vi "GT Active Scheduler wSubset Standalone.vi"() -> ()   [LabVIEW 2013, in "Scheduler.lvclass"]
uses:
  Scheduler.lvclass
  OSSP_Problem.lvclass
  Operation Selection Rule from Subset to Schedule.ctl
  Prins FIFO Scheduler Methods and Controls/Controls/Prins FIFO Scheduler Result Cluster.ctl
  OSSP_Problem.lvclass/OSSP_Problem.ctl
  Operation to Machine Job Tuple.vi
  GT Find Subset of Operations.vi
  Select Operation to Schedule Based on Rule.vi
  OSSP_Problem_Class/Getters/Read Due Dates.vi
  <vilib>/dlg_ctls.llb/Space Constant.vi
  <vilib>/Heliosphere Research LLC/Advanced Plotting Toolkit/api_core/New.vi
  <vilib>/Heliosphere Research LLC/Advanced Plotting Toolkit/api_annotations/XLabel.vi
  <vilib>/Heliosphere Research LLC/Advanced Plotting Toolkit/api_figure/YTicks.vi
  <vilib>/Heliosphere Research LLC/Advanced Plotting Toolkit/api_figure/Grids.vi
  <vilib>/Heliosphere Research LLC/Advanced Plotting Toolkit/api_core/View.vi
  <vilib>/Heliosphere Research LLC/Advanced Plotting Toolkit/api_core/Close.vi
  <vilib>/Heliosphere Research LLC/Advanced Plotting Toolkit/api_figure/Limits.vi
  <vilib>/Heliosphere Research LLC/Advanced Plotting Toolkit/api_annotations/Rectangle.vi
  <vilib>/Heliosphere Research LLC/Advanced Plotting Toolkit/api_annotations/Text.vi
panel:
  out "Graph Out":picture
  out "Ordered Schedule Out":u16[](array[numeric])
  in  "Problem Type":enum16{"Taillard", "Brucker", "Gueret Prins"}(ring)
  in  "Instance Number for Taillard":dbl
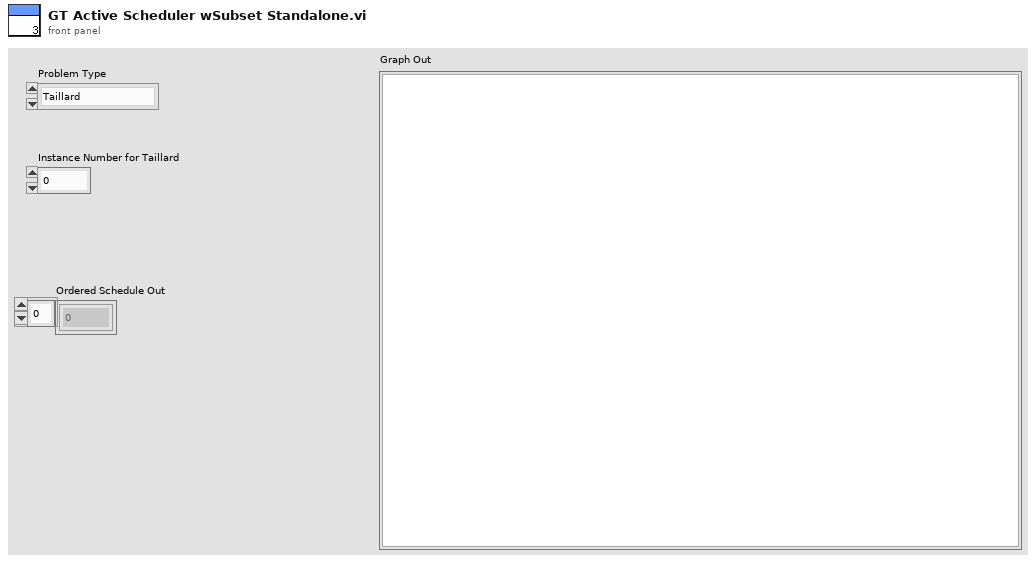
[diagram p1: front panel]
types:
  T1 = typedef "Scheduler.lvclass/Prins FIFO Scheduler Result Cluster.ctl" = cluster{"Start Times":u16[][], "Completion Times":u16[][], "Processing Times":u16[][]}
  T2 = typedef "Scheduler.lvclass/Operation Selection Rule from Subset to Schedule.ctl" = enum16{"First Operation in Order", "SPT", "EDD", "MDD"}
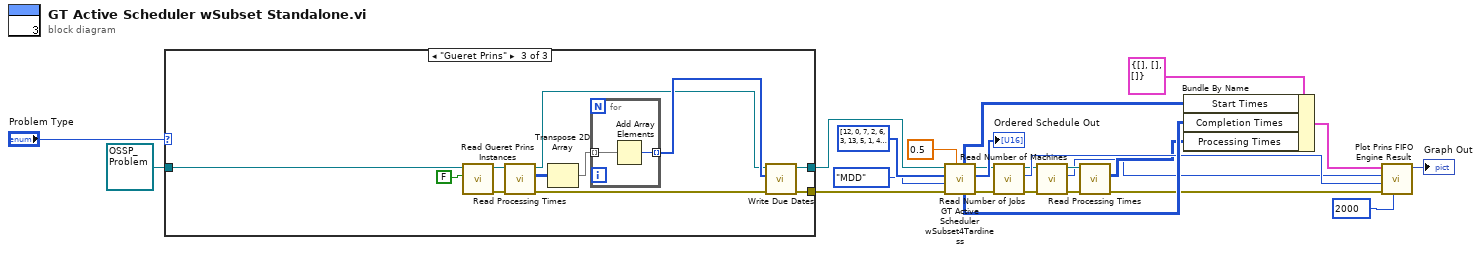
[diagram p0: block diagram]
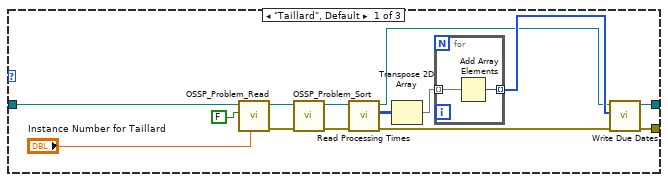
[diagram p2: hidden frame]
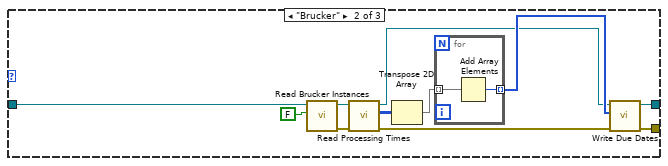
[diagram p3: hidden frame]
diagram:
  n1 = case shown="\"Gueret Prins\"" "Problem Type" {
    tunnel: refnum<class "OSSP_Problem.lvclass"> refnum ("OSSP_Problem.lvclass") -> [w38 w51 w64]
    tunnel: [w31 w46 w59] -> w22
    tunnel: [w30 w47 w60] -> w21
    frame "Taillard", Default {
      n2 = call "OSSP_Problem_Read.vi"("Instance Number"="Instance Number for Taillard", "Auto Mode"=FALSE, "OSSP_Problem.lvclass In"=w38) -> ("error out"=w35:errorcluster, "OSSP_Problem.lvclass Out"=w36:refnum<class "OSSP_Problem.lvclass">)  [unwired: 7 in]
      n3 = call "OSSP_Problem_Sort.vi"("error in (no error)"=w35, "OSSP_Problem.lvclass In"=w36) -> ("error out"=w33:errorcluster, "OSSP_Problem.lvclass Out"=w32:refnum<class "OSSP_Problem.lvclass">)  [unwired: 8 in]
      n4 = call "Read Processing Times.vi"("error in (no error)"=w33, "OSSP_Problem in"=w32) -> ("error out"=w25:errorcluster, "Processing Times"=w28:u16[][], "OSSP_Problem out"=w26:refnum<class "OSSP_Problem.lvclass">)  [unwired: 7 in]
      n5 = Transpose 2D Array(2D array=w28) -> (transposed array=w29:u16[][])
      n6 = for {
        tunnel: w29 -> [w40] mode=indexing
        tunnel: [w39] -> w27 mode=indexing
        n7 = Add Array Elements(numeric array=w40) -> (sum=w39:u16)
      }
      n8 = call "Write Due Dates.vi"("error in (no error)"=w25, "Due Dates"=w27, "OSSP_Problem in"=w26) -> ("error out"=w30:errorcluster, "OSSP_Problem out"=w31:refnum<class "OSSP_Problem.lvclass">)  [unwired: 7 in]
    }
    frame "Brucker" {
      n9 = call "Read Brucker Instances.vi"("Auto Mode"=FALSE, "OSSP_Problem in"=w51) -> ("error out"=w48:errorcluster, "OSSP_Problem out"=w49:refnum<class "OSSP_Problem.lvclass">)  [unwired: 8 in]
      n10 = call "Read Processing Times.vi"("error in (no error)"=w48, "OSSP_Problem in"=w49) -> ("error out"=w41:errorcluster, "Processing Times"=w44:u16[][], "OSSP_Problem out"=w42:refnum<class "OSSP_Problem.lvclass">)  [unwired: 7 in]
      n11 = Transpose 2D Array(2D array=w44) -> (transposed array=w45:u16[][])
      n12 = for {
        tunnel: w45 -> [w53] mode=indexing
        tunnel: [w52] -> w43 mode=indexing
        n13 = Add Array Elements(numeric array=w53) -> (sum=w52:u16)
      }
      n14 = call "Write Due Dates.vi"("error in (no error)"=w41, "Due Dates"=w43, "OSSP_Problem in"=w42) -> ("error out"=w47:errorcluster, "OSSP_Problem out"=w46:refnum<class "OSSP_Problem.lvclass">)  [unwired: 7 in]
    }
    frame "Gueret Prins" {
      n15 = call "Read Gueret Prins Instances.vi"("Auto Mode"=FALSE, "OSSP_Problem in"=w64) -> ("error out"=w61:errorcluster, "OSSP_Problem out"=w62:refnum<class "OSSP_Problem.lvclass">)  [unwired: 8 in]
      n16 = call "Read Processing Times.vi"("error in (no error)"=w61, "OSSP_Problem in"=w62) -> ("error out"=w54:errorcluster, "Processing Times"=w57:u16[][], "OSSP_Problem out"=w55:refnum<class "OSSP_Problem.lvclass">)  [unwired: 7 in]
      n17 = Transpose 2D Array(2D array=w57) -> (transposed array=w58:u16[][])
      n18 = for {
        tunnel: w58 -> [w66] mode=indexing
        tunnel: [w65] -> w56 mode=indexing
        n19 = Add Array Elements(numeric array=w66) -> (sum=w65:u16)
      }
      n20 = call "Write Due Dates.vi"("error in (no error)"=w54, "Due Dates"=w56, "OSSP_Problem in"=w55) -> ("error out"=w60:errorcluster, "OSSP_Problem out"=w59:refnum<class "OSSP_Problem.lvclass">)  [unwired: 7 in]
    }
  }
  n21 = call "GT Active Scheduler wSubset4Tardiness.vi"("Lambda"=0.5, "error in (no error)"=w21, "Operation Selection Rule"=Operation_Selection_Rule_from_Subset_to_Schedule."MDD", "Schedule In"=u16[] [12, 0, 7, 2, 6, 3, 13, 5, 1, 4, 14, 11, 10, 15, 8, 9], "OSSP_Problem.lvclass"=w22) -> ("error out"=w16:errorcluster, "Ordered Schedule Out"=→"Ordered Schedule Out":u16[], "OSSP_Problem out"=w15:refnum<class "OSSP_Problem.lvclass">, "Completion Times"=w14:u16[][], "Start Times"=w17:u16[][])  [unwired: 1 in, 1 out]
  n22 = call "Read Number of Jobs.vi"("error in (no error)"=w16, "OSSP_Problem in"=w15) -> ("error out"=w8:errorcluster, "Number of Jobs"=w9:i32, "OSSP_Problem out"=w5:refnum<class "OSSP_Problem.lvclass">)  [unwired: 7 in]
  n23 = call "Read Number of Machines.vi"("error in (no error)"=w8, "OSSP_Problem in"=w5) -> ("error out"=w7:errorcluster, "Number of Machines"=w2:i32, "OSSP_Problem out"=w4:refnum<class "OSSP_Problem.lvclass">)  [unwired: 7 in]
  n24 = call "Read Processing Times.vi"("error in (no error)"=w7, "OSSP_Problem in"=w4) -> ("error out"=w6:errorcluster, "Processing Times"=w3:u16[][])  [unwired: 7 in, 1 out]
  n25 = Bundle By Name(cluster=T1 {"Start Times"=[], "Completion Times"=[], "Processing Times"=[]} ("FIFO Results"), "Start Times"=w17, "Completion Times"=w14, "Processing Times"=w3) -> (w12:T1)
  n26 = call "Plot Prins FIFO Engine Result.vi"("Plot Max Value"=2000, "error in (no error)"=w6, "Number of Jobs"=w9, "Number of Machines"=w2, "FIFO Results"=w12) -> ("Graph Out"=→"Graph Out":picture)  [unwired: 5 in, 1 out]
